vi "3array2number.vi"(3 "Index":i32, 4 "Array3":u8[](array[numeric]), 5 "Array 2":u8[](array[numeric]), 6 "Array1":u8[](array[numeric])) -> (0 "VAL3":u8, 1 "VAL2":u8, 2 "VAL1":u8)   [LabVIEW 2018]
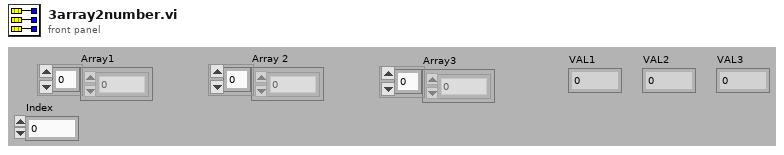
[diagram p1: front panel]
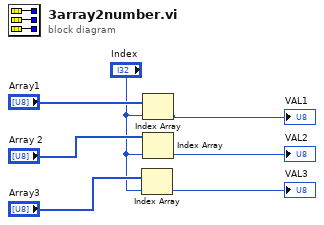
[diagram p0: block diagram]
diagram:
  n1 = Index Array(array="Array3", index="Index") -> (element=→"VAL3":u8)
  n2 = Index Array(array="Array1", index="Index") -> (element=→"VAL1":u8)
  n3 = Index Array(array="Array 2", index="Index") -> (element=→"VAL2":u8)
